vi "DELETE.vi"(6 "timeout (10000)":i32=10000, 7 "output file":path=path "", 8 "error in (no error)":errorcluster, 10 "url":string, 11 "HTTP Client Base in":refnum<class "HTTP Client Base.lvclass">) -> (0 "error out":errorcluster, 1 "body":string, 2 "headers":string, 3 "HTTP Client Base out":refnum<class "HTTP Client Base.lvclass">)   [LabVIEW 2021, in "HTTP Client Base.lvclass"]
uses:
  HTTP Client Base.lvclass
  HTTP Client Base.lvclass/HTTP Client Base.ctl
  <vilib>/httpClient/LabVIEWHTTPClient.lvlib
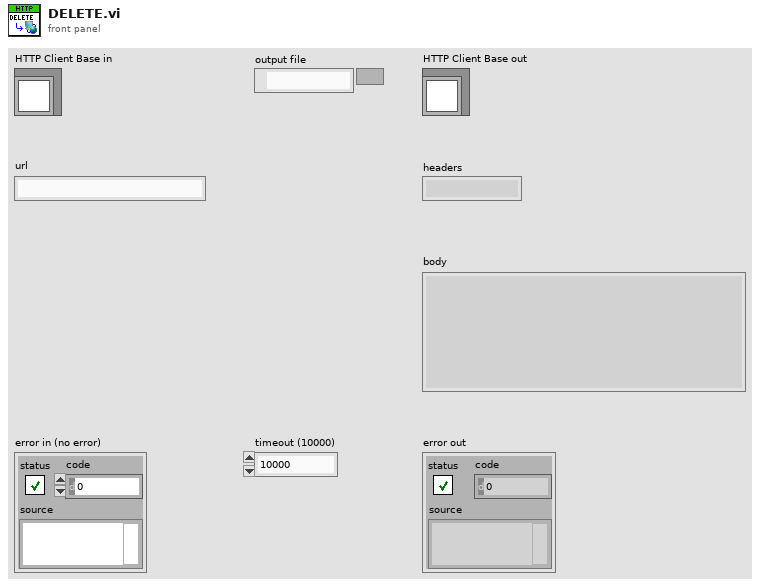
[diagram p1: front panel]
types:
  T1 = typedef "LabVIEWHTTPClient.lvlib/ClientHandle.ctl" = refnum<k1>
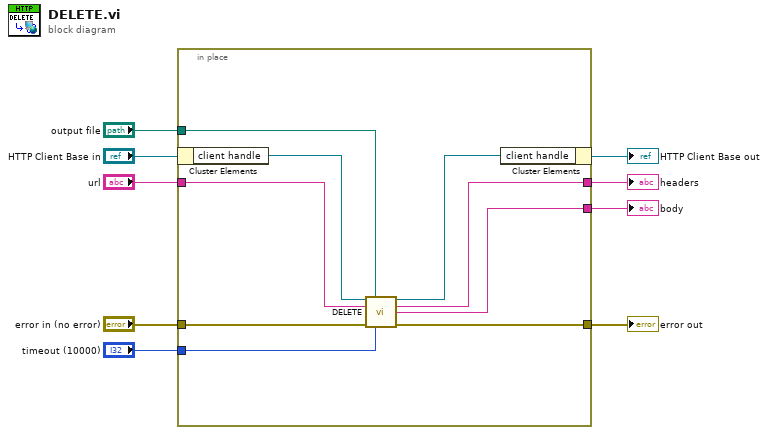
[diagram p0: block diagram]
diagram:
  n1 = in-place {
    in-place-border: "error in (no error)" -> [w18]
    in-place-border: [w17] -> w7
    in-place-border: "output file" -> [w14]
    in-place-border: "url" -> [w13]
    in-place-border: "timeout (10000)" -> [w12]
    in-place-border: [w11] -> w2
    in-place-border: [w10] -> w1
    n2 = in-place-cluster #1("HTTP Client Base in") -> ("client handle"=w16:T1)
    n3 = call <vilib>:"DELETE.vi"("client handle"=w16, "output file"=w14, "url"=w13, "error in (no error)"=w18, "timeout (10000)"=w12) -> ("client handle out"=w15:T1, "headers"=w11:string, "body"=w10:string, "error out"=w17:errorcluster)  [unwired: 7 in]
    n4 = in-place-cluster #1("client handle"=w15) -> (→"HTTP Client Base out":refnum<class "HTTP Client Base.lvclass">)
  }
  "error out" <- w7
  "headers" <- w2
  "body" <- w1
